vi "NTP Sync.vi"(8 "error in (no error)":errorcluster, 11 "Time Server IP":string="132.163.4.102") -> (0 "error out":errorcluster, 2 "Time Set?":bool, 3 "Time Set":timestamp)   [LabVIEW 2017]
uses:
  <vilib>/Utility/miscctls.llb/LVDateTimeRec.ctl
  <vilib>/nisyscfg/nisyscfg.lvlib
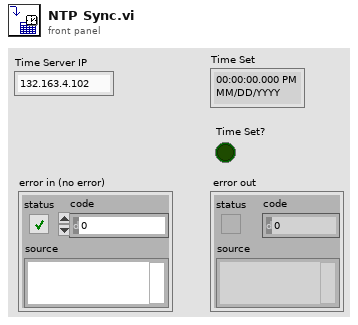
[diagram p1: front panel]
types:
  T1 = typedef "LVDateTimeRec.ctl" = cluster{"fractional second":dbl, "second":i32, "minute":i32, "hour":i32, "day of month":i32, "month":i32, "year":i32, "day of week":i32, "day of year":i32, "DST":i32}
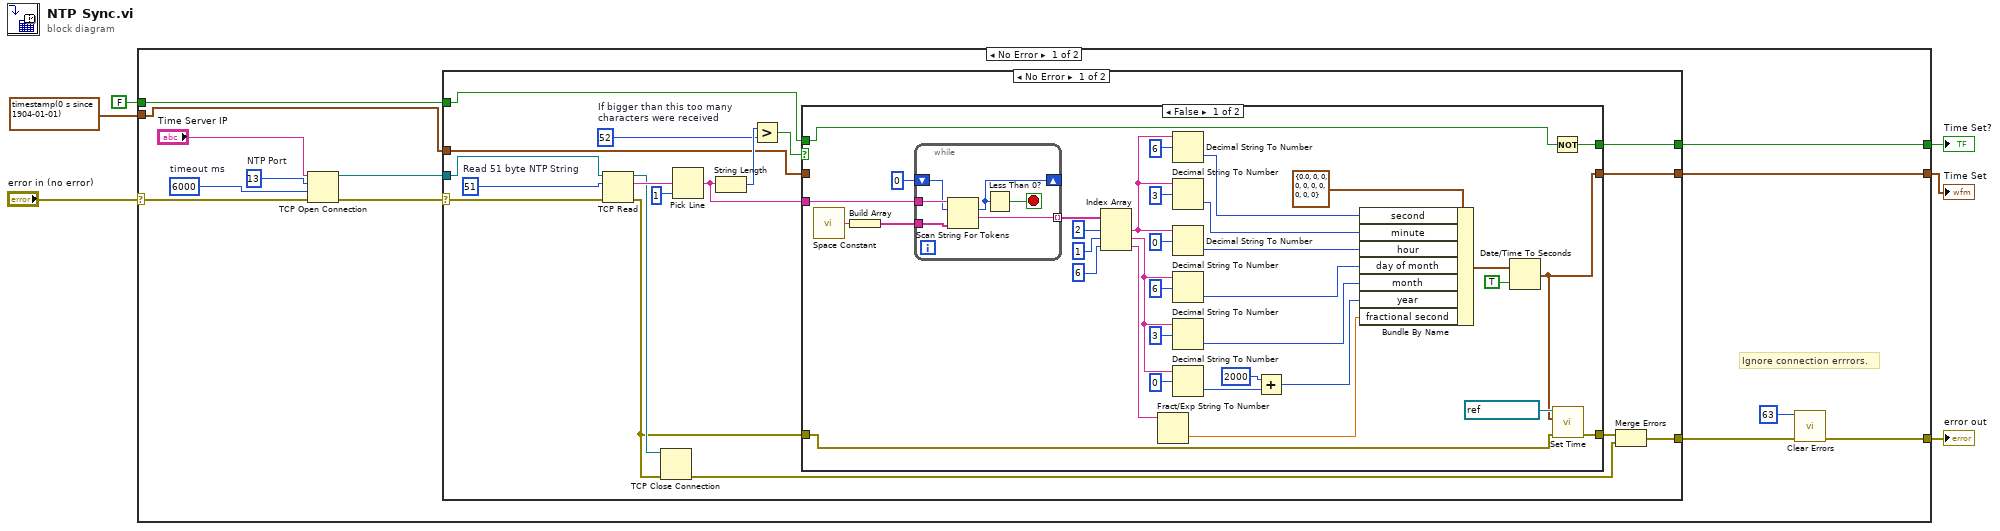
[diagram p0: block diagram]
diagram:
  n1 = case shown="No Error" "error in (no error)" {
    selector: "error in (no error)" -> [w13 w87]
    tunnel: [w9 w87] -> w6
    tunnel: [w14 w86] -> w3
    tunnel: timestamp(0 s since 1904-01-01) ("Time Set") -> [w12 w86]
    tunnel: [w11 w85] -> w2
    tunnel: FALSE -> [w10 w85]
    frame No Error {
      w17 = 6000  # timeout ms
      w18 = u16 13  # NTP Port
      # "Ignore connection errrors."
      n2 = TCP Open Connection(address="Time Server IP", remote port or service name=w18, timeout ms (60000)=w17, error in (no error)=w13) -> (connection ID=w19:refnum<k5>, error out=w16:errorcluster)  [unwired: 1 in]
      n3 = case shown="No Error" w16 {
        selector: w16 -> [w29 w84]
        tunnel: w19 -> [w36 _]
        tunnel: [w24 w84] -> w8
        tunnel: [w26 w83] -> w14
        tunnel: w12 -> [w22 w83]
        tunnel: [w21 w82] -> w11
        tunnel: w10 -> [w20 w82]
        frame No Error {
          w30 = 52  # If bigger than this too many characters were received
          w37 = 51  # Read 51 byte NTP String
          n4 = TCP Read(connection ID=w36, bytes to read=w37, error in (no error)=w29) -> (connection ID out=w28:refnum<k5>, data out=w34:string, error out=w25:errorcluster)  [unwired: 2 in]
          n5 = TCP Close Connection(connection ID=w28, error in (no error)=w25) -> (error out=w23:errorcluster)  [unwired: 1 in, 1 out]
          n6 = Pick Line(multi-line string=w34, line index=1) -> (output string=w33:string)  [unwired: 1 in]
          n7 = String Length(string=w33) -> (length=w32:i32)
          n8 = Greater?(x=w32, y=w30) -> (0:w31:bool)
          n9 = case shown="False" w31 {
            tunnel: w33 -> [w43 _]
            tunnel: w25 -> [w54 w81]
            tunnel: [w53 w81] -> w27
            tunnel: [w45 w80] -> w26
            tunnel: w22 -> [_ w80]
            tunnel: [w39 w79] -> w21
            tunnel: w20 -> [w38 w79]
            frame False {
              n10 = call <vilib>:"Space Constant.vi"() -> ("String"=w42:string)
              n11 = Build Array(w42) -> (w41:string[])
              n12 = while {
                tunnel: w43 -> [w78]
                shift-right: [w73] -> _
                shift-left: 0 ("offset past token") -> [w77]
                tunnel: [w76] -> w44 mode=indexing
                tunnel: w41 -> [w75]
                stop <- w74 stop-if-true
                n13 = Scan String For Tokens(6:w75, 8:w77, 9:w78) -> (1:w76:string, 2:w73:i32)  [unwired: 3 in, 2 out]
                n14 = Less Than 0?(x=w73) -> (x < 0?=w74:bool)
              }
              n15 = Index Array(array=w44, index #1=2 ("index"), index #2=1 ("index"), index #3=6 ("index")) -> (element #1=w49:string, element #2=w48:string, element #3=w47:string)
              n16 = Fract/Exp String To Number(string=w47) -> (number=w70:dbl)  [unwired: 3 in, 1 out]
              n17 = Decimal String To Number(string=w49, offset=6) -> (number=w59:i32)  [unwired: 1 in, 1 out]
              n18 = Decimal String To Number(string=w49, offset=3) -> (number=w63:i32)  [unwired: 1 in, 1 out]
              n19 = Decimal String To Number(string=w49, offset=0) -> (number=w61:i32)  [unwired: 1 in, 1 out]
              n20 = Decimal String To Number(string=w48, offset=6) -> (number=w65:i32)  [unwired: 1 in, 1 out]
              n21 = Decimal String To Number(string=w48, offset=3) -> (number=w67:i32)  [unwired: 1 in, 1 out]
              n22 = Decimal String To Number(string=w48, offset=0) -> (number=w69:i32)  [unwired: 1 in, 1 out]
              n23 = Add(x=2000, y=w69) -> (x+y=w71:i32)
              n24 = Bundle By Name(cluster=T1 {"fractional second"=0.0, "second"=0, "minute"=0, "hour"=0, "day of month"=0, "month"=0, "year"=0, "day of week"=0, "day of year"=0, "DST"=0} ("date time rec"), "second"=w59, "minute"=w63, "hour"=w61, "day of month"=w65, "month"=w67, "year"=w71, "fractional second"=w70) -> (w56:T1)
              n25 = Date/Time To Seconds(1:TRUE ("is UTC (F)"), 2:w56) -> (0:w45:timestamp)
              n26 = Not(x=w38) -> (.not. x?=w39:bool)
              n27 = call <vilib>:"Set Time.vi"("error in (no error)"=w54, "Time"=w45, "Session in (localhost)"=refnum<k21> "localhost" ("session in (localhost)")) -> ("error out"=w53:errorcluster)  [unwired: 5 in, 3 out]
            }
            frame True {
            }
          }
          n28 = Merge Errors(w27, w23) -> (w24:errorcluster)
        }
        frame Error {
          # "Network Error Do Nothing"
        }
      }
      n29 = call <vilib>:"Clear Errors.vi"("error in (no error)"=w8, "specific error code to clear (0: all)"=63) -> ("error out"=w9:errorcluster)  [unwired: 4 in, 1 out]
    }
    frame Error {
    }
  }
  "error out" <- w6
  "Time Set" <- w3
  "Time Set?" <- w2
